vi "De-NaNArray.vi"(3 "ArrayIn":dbl[](array[numeric])) -> (0 "GoodFraction":dbl, 1 "de-NaN-dArrayOut":dbl[](array[numeric]))   [LabVIEW 2013]
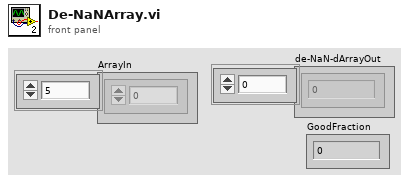
[diagram p1: front panel]
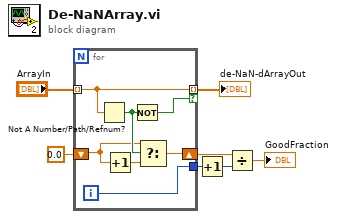
[diagram p0: block diagram]
diagram:
  n1 = for {
    tunnel: "ArrayIn" -> [w14] mode=indexing
    tunnel: [w14] -> w6 mode=indexing if=w13
    shift-right: [w12] -> w5
    shift-left: 0.0 -> [w9]
    tunnel: [w8] -> w4
    i -> [w8]
    n2 = Not A Number/Path/Refnum?(number/path/refnum=w14) -> (NaN/Path/Refnum?=w11:bool)
    n3 = Increment(x=w9) -> (x+1=w10:dbl)
    n4 = Not(x=w11) -> (.not. x?=w13:bool)
    n5 = Select(t=w9, s=w11, f=w10) -> (s? t:f=w12:dbl)
  }
  "de-NaN-dArrayOut" <- w6
  n6 = Increment(x=w4) -> (x+1=w3:i32)
  n7 = Divide(x=w5, y=w3) -> (x/y=→"GoodFraction":dbl)
